vi "Loop_SM.vi"() -> ()   [LabVIEW 2017, in "Overlords.lvlib"]
uses:
  Overlords.lvlib
  ENUM _Overloard Shooter States.ctl
  VisionSystem/Enum_ Field Targets.ctl
  VisionSystem/VisionSystem.lvlib
  MechamumDrive/Enum_SM Cmd Select.ctl
  MechamumDrive/MechamunDrive.lvlib
  MechamumDrive/Cluster_CMD to SM Data.ctl
  MechamumDrive/Global_CMD to SM Data.vi
  MechamumDrive/Global_SM Out Data.vi
  Globals/Global_Hopper Statis.vi
  Hopper/Hopper System.lvlib
  ENUM_Overloard State.ctl
  ENUM_Overloard Gear States.ctl
  Sonar/Global_HW_Data Out.vi
  Sonar/Sonar.lvlib
  MechamumDrive/Global_HW_Status Out.vi
  Gear/Global_HW_Data Out.vi
  Gear/Gear.lvlib
  ENUM_Overloard Climb States.ctl
  Climber/Global_SM_Data Out.vi
  Climber/Climber.lvlib
  Climber/ENUM_SM Cmd Select.ctl
  Climber/Global_CMD to SM Data.vi
  VisionSystem/Global_CMD Data.vi
  VisionSystem/Cluster_CMD to Vision.ctl
  VisionSystem/Global_Vision Status.vi
  Shooter/Global_CMD to SM Data.vi
  Shooter/Shooter.lvlib
  Shooter/ENUM_CMD Select.ctl
  Shooter/Cluster_CMD to SM Data.ctl
  Globals/Global_CMD to SM Data.vi
  Hopper/ENUM_Firing_State.ctl
  Hopper/Cluster_CMD to SM Data.ctl
  Global_CMD Data.vi
  Global_SM_Data Out.vi
panel:
  in  "stop":bool
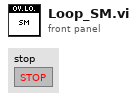
[diagram p1: front panel]
types:
  T1 = typedef "Hopper System.lvlib/ENUM_Firing_State.ctl" = enum16{"No Fireing", "Rapid Fire", "Shotgun Fireing"}
  T2 = typedef "Hopper System.lvlib/Cluster_CMD to SM Data.ctl" = cluster{"Enable Loading":bool, "Disable Loading":bool, "Fireing State":T1, "Time Limit Loading":dbl, "Time Limit Rapid":dbl, "Rapid Fire Shot Limit":i32, "Shotgun Fire Shot Limit":i32}
  T3 = typedef "Shooter.lvlib/ENUM_CMD Select.ctl" = enum16{"Stop", "Manual VBus", "Encoder Hood Only", "Encoder Wheel Only", "Encoder Both"}
  T4 = typedef "Shooter.lvlib/Cluster_CMD to SM Data.ctl" = cluster{"Select":T3, "Wheel VBus":dbl, "Wheel RPM":dbl, "Hood VBus":dbl, "Hood Position":dbl}
  T5 = typedef "MechamunDrive.lvlib/Enum_SM Cmd Select.ctl" = enum16{"No Command", "Halt", "Manual Keep Rotation", "Manual", "Track Front", "Track Rotation", "Track Lateral", "Track Vision Lat", "Track Vision Rot", "Strafe Right", "Strafe Left"}
  T6 = typedef "MechamunDrive.lvlib/Cluster_CMD to SM Data.ctl" = cluster{"CMDMODE":T5, "X":dbl, "Y":dbl, "Rotation":dbl, "Auto Angle":dbl, "Speed Divider":dbl, "Use Gyro":bool, "Target Distance":dbl}
  T7 = typedef "Climber.lvlib/ENUM_SM Cmd Select.ctl" = enum16{"Stop", "Auto Climb", "Manual", "No Command"}
  T8 = typedef "Overlords.lvlib/ENUM_Overloard State.ctl" = enum16{"Idle", "High Shot", "Low Shot", "Place Gear", "Climb"}
  T9 = typedef "Overlords.lvlib/ENUM _Overloard Shooter States.ctl" = enum16{"Startup", "Idle", "Locate Target", "Wait To Be in Position", "Shooting", "Complete"}
  T10 = typedef "VisionSystem.lvlib/Cluster_CMD to Vision.ctl" = cluster{"CMD_Target":T11}
  T11 = typedef "VisionSystem.lvlib/Enum_ Field Targets.ctl" = enum16{"Boiler (USB 0)", "Rope (USB 1)"}
  T12 = typedef "Overlords.lvlib/ENUM_Overloard Gear States.ctl" = enum16{"Startup", "Idle", "Detect Target", "Verticle Track (Sonar)", "Encoder Setup", "Verticle Track (Encoder)", "Gear Present", "Gear Present Counter", "Verticle Backword Track", "Complete"}
  T13 = typedef "Overlords.lvlib/ENUM_Overloard Climb States.ctl" = enum16{"Startup", "Idle", "Check Time", "Check Statis", "Complete"}
  T14 = typedef "Overlords.lvlib/Cluster_CMD to SM Data.ctl" = cluster{"Overloard State":T8, "Match Info":T15, "Firing State":T1, "Gear wait till pullback (seconds)":dbl}
  T15 = typedef "WPI_DriverStationMatch Info.ctl" = cluster{"Autonomous Elapsed Seconds":dbl, "TeleOp Elapsed Seconds":dbl, "Disabled Elapsed Seconds":dbl, "Visited Autonomous":bool, "Visited TeleOp":bool, "Visited Disabled":bool, "Autonomous Settings":cluster{"Autonomous Style":enum16{"Iterative", "Independent"}, "VI Refnum":refnum<vi>}}
  T16 = typedef "Overlords.lvlib/Cluster_SM Status.ctl" = cluster{"Task Complete":bool, "Current Overlord State":T8, "Wanted State":T8, "Overloard Shooter States":T9, "Overlord Gear State":T12, "Overlord Climber State":T13}
  T17 = typedef "Climber.lvlib/Cluster_Cmd to SM Data.ctl" = cluster{"Climber Command Mode":T7}
  T18 = typedef "VisionSystem.lvlib/Cluster_Vision Status.ctl" = cluster{"Target Found":bool, "Target":T11, "Pixels to Center":dbl, "Vision Distance Center (in)":dbl, "Angle Distance Center (in)":dbl}
  T19 = typedef "MechamunDrive.lvlib/Cluster_SM Status.ctl" = cluster{"Drive Cmd":T5, "Complete":bool}
  T20 = typedef "MechamunDrive.lvlib/Cluster_HW Status.ctl" = cluster{"BL":T21, "BR":T21, "FL":T21, "FR":T21}
  T21 = typedef "Cluster_SRX Status With Encoder.ctl" = cluster{"VBus ":dbl, "Module Enabled":bool, "Closed Loop Error":dbl, "Sensor Pos":dbl, "Sensor Vel":dbl, "Current":dbl, "Brake is Enabled":bool, "Encoder Pos":dbl, "Encoder Vel":dbl, " APin":bool, "B Pin":bool, "Bat Voltage":dbl, "Profile Slot":dbl}
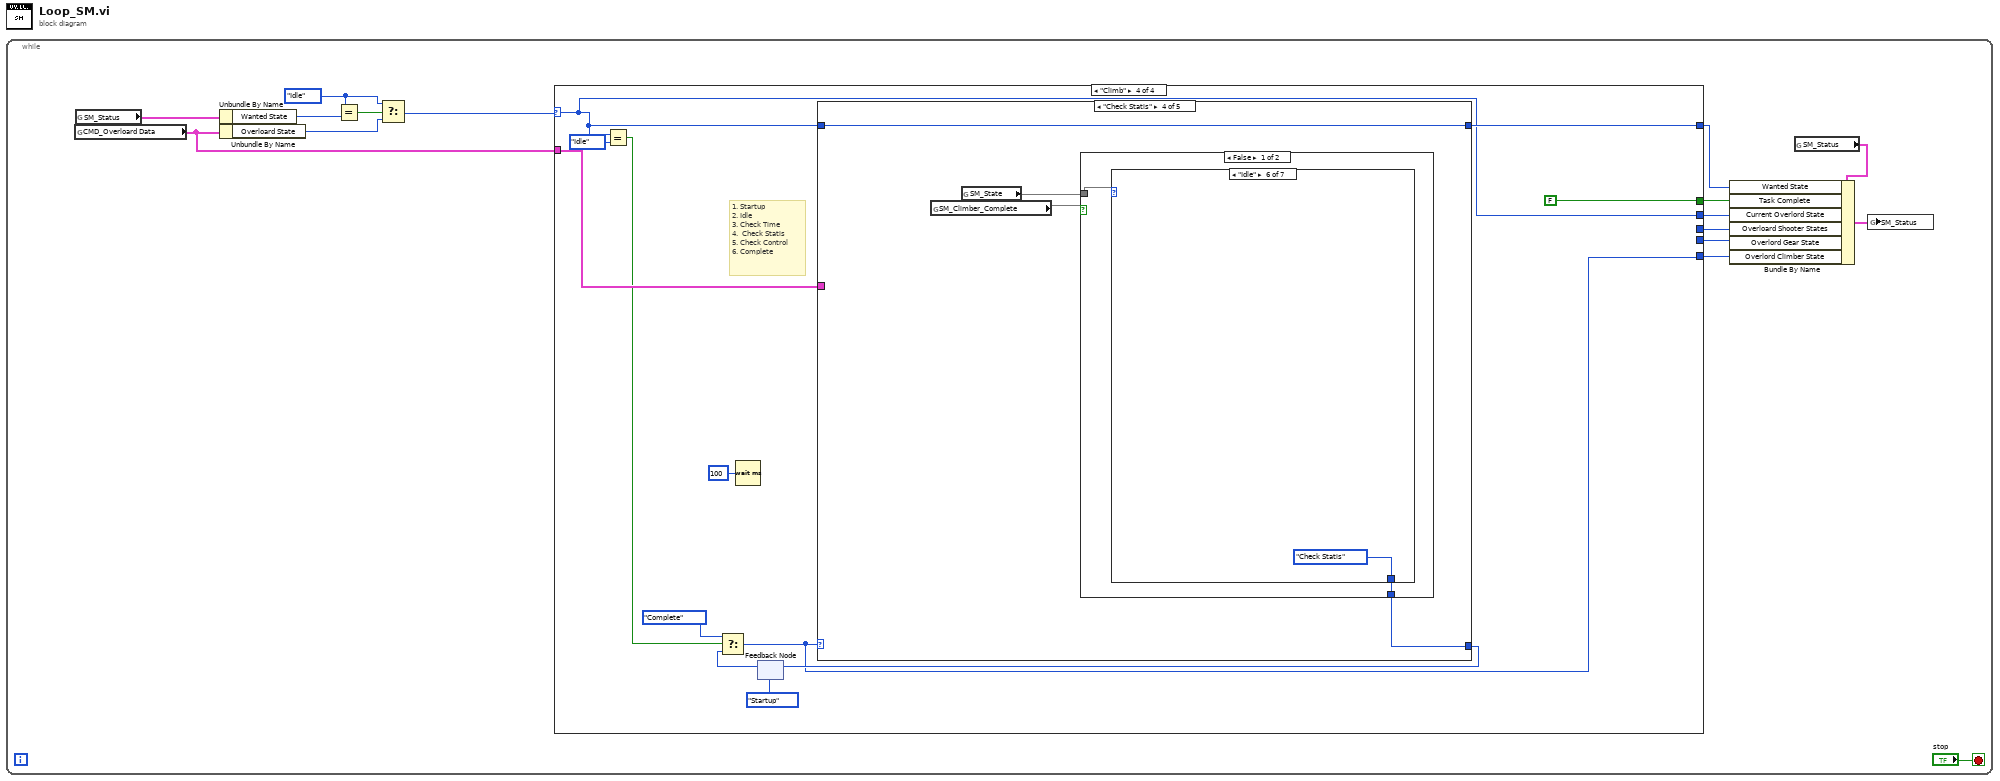
[diagram p0: block diagram]
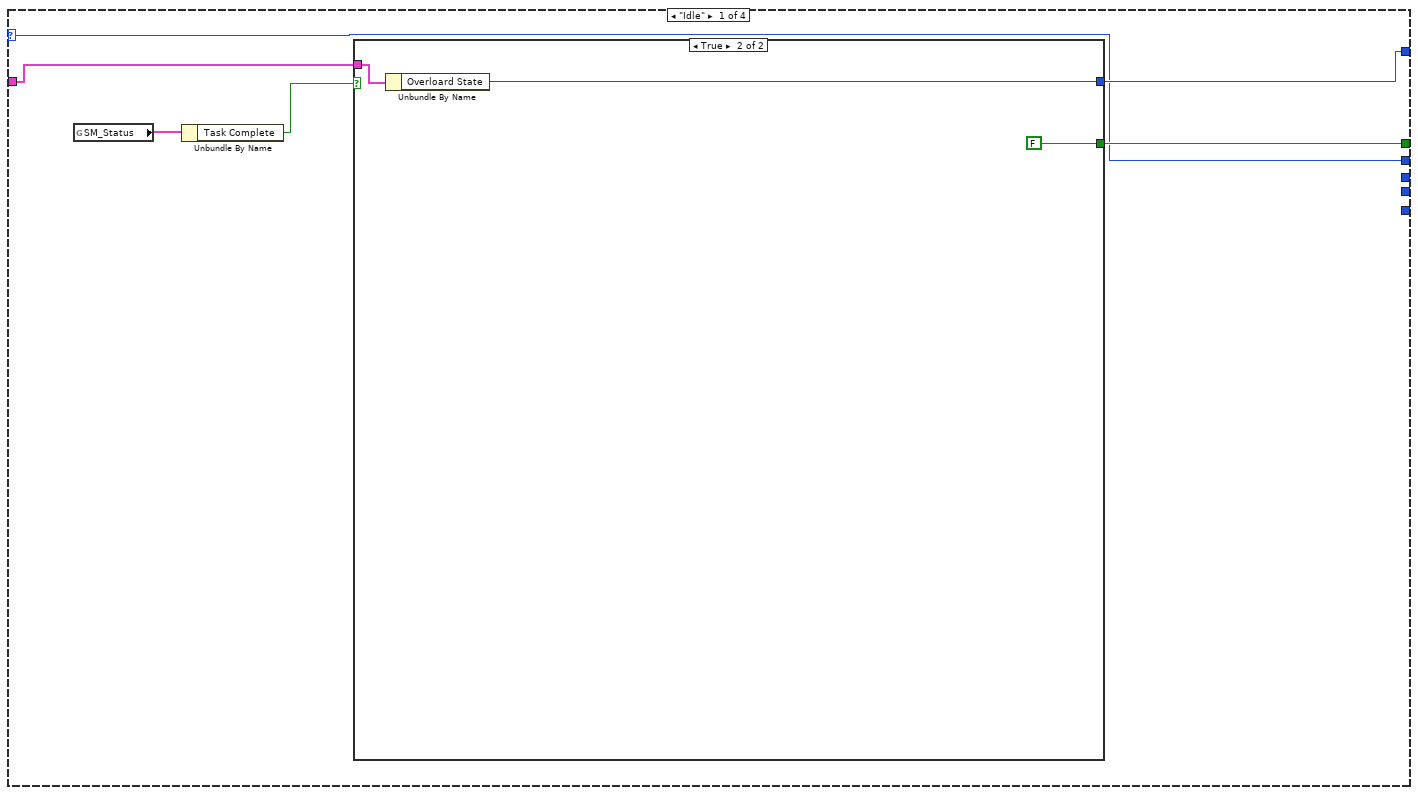
[diagram p2: hidden frame]
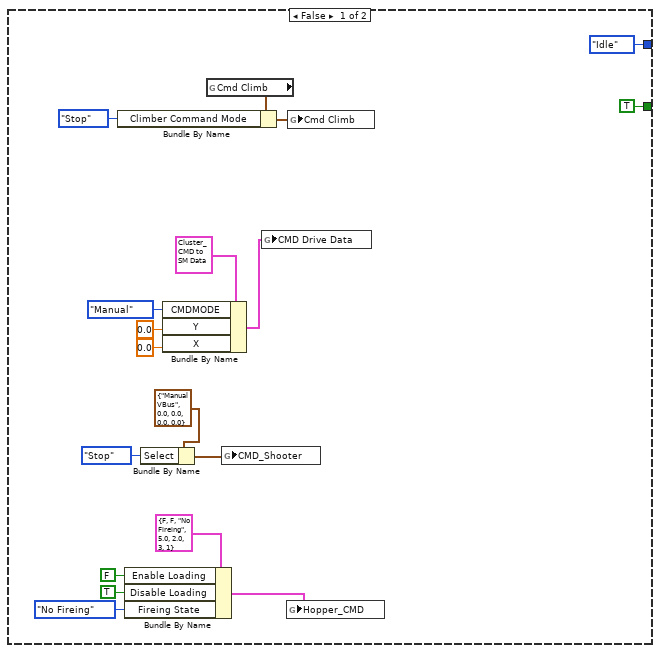
[diagram p3: hidden frame]
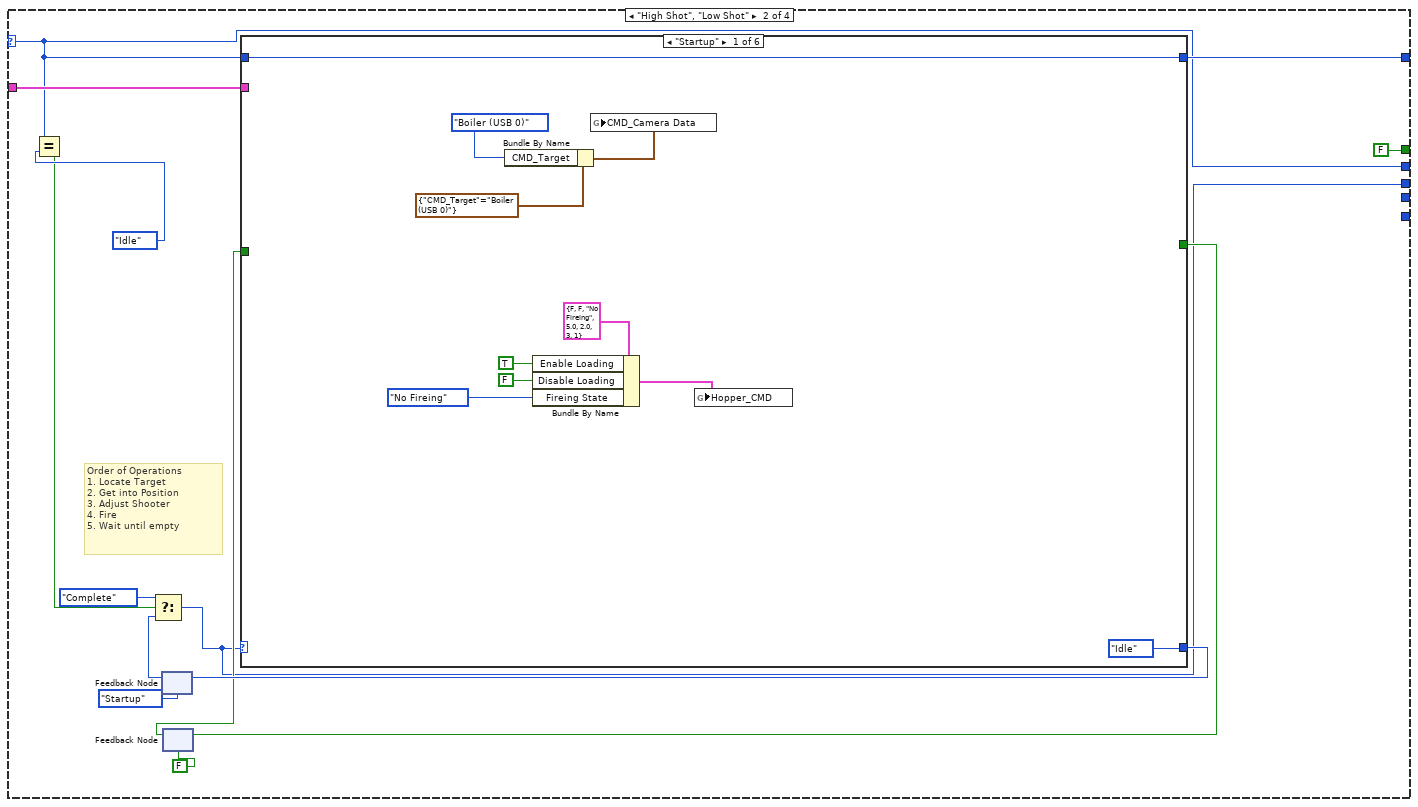
[diagram p4: hidden frame]
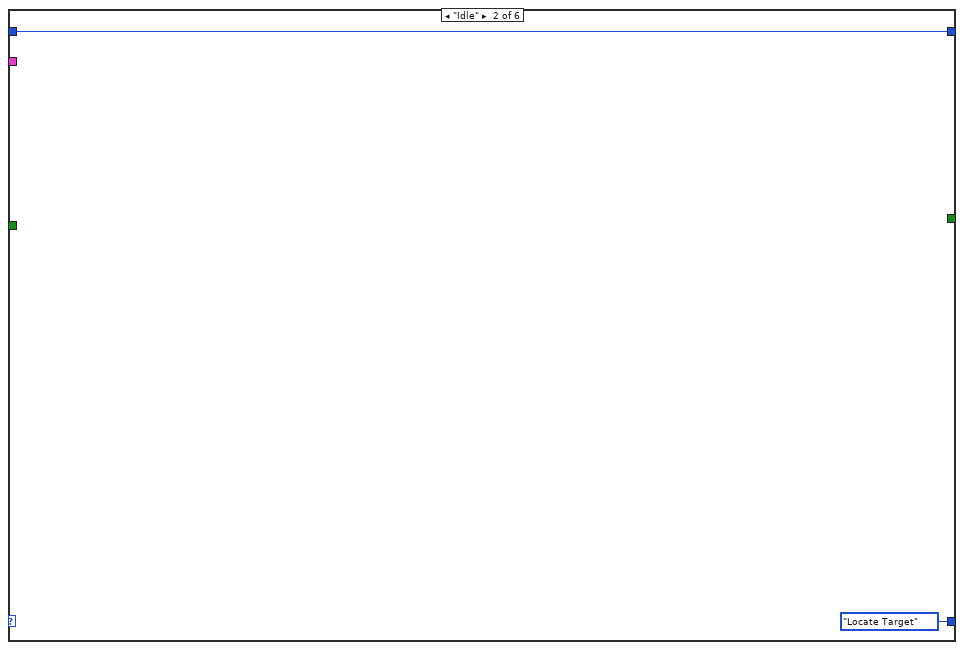
[diagram p5: hidden frame]
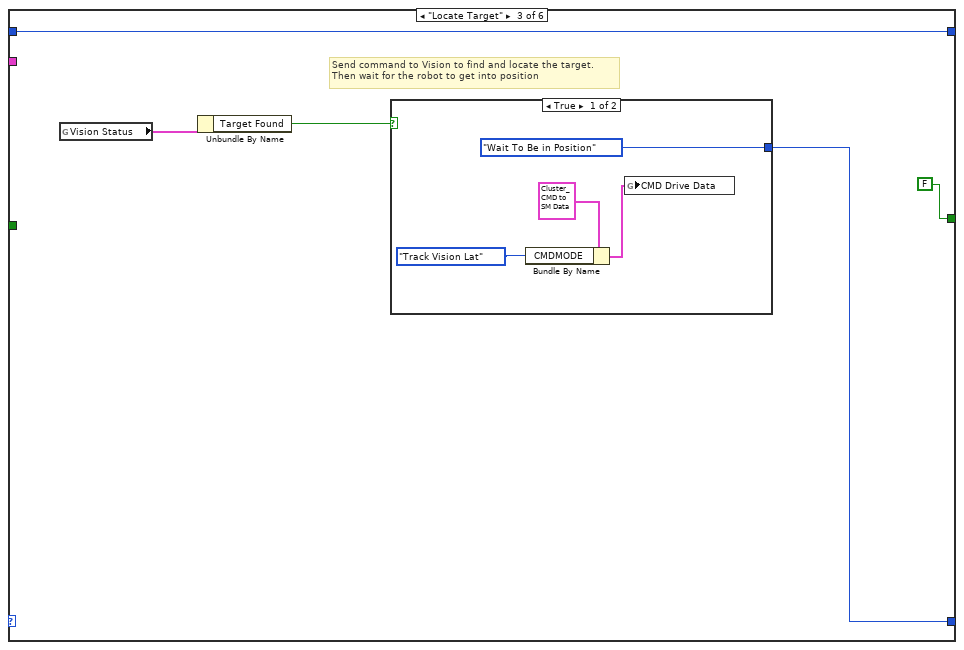
[diagram p6: hidden frame]
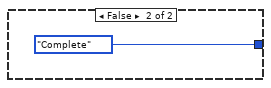
[diagram p7: hidden frame]
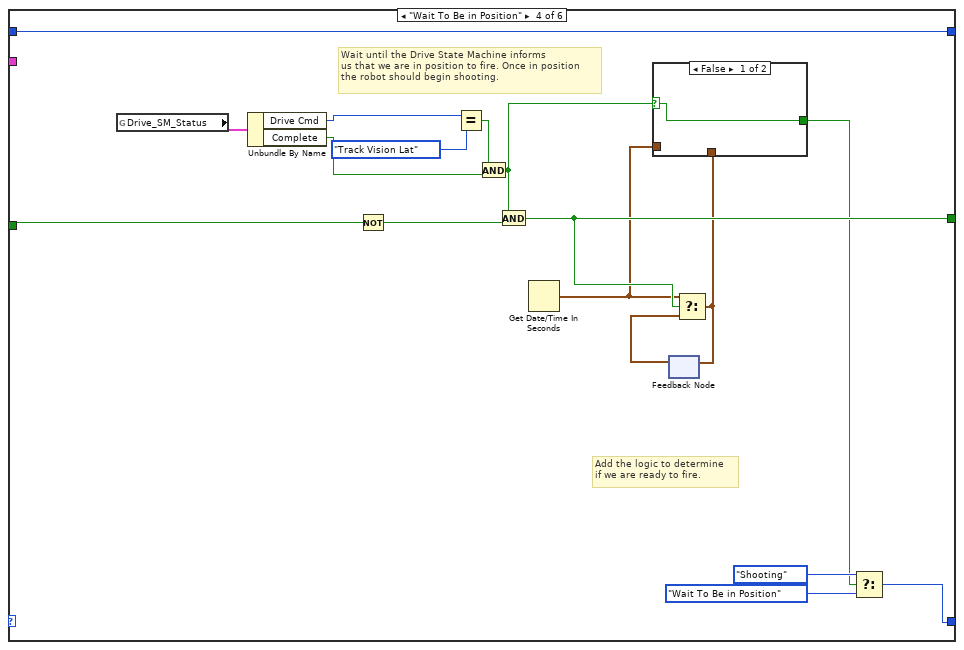
[diagram p8: hidden frame]
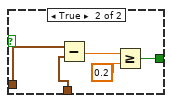
[diagram p9: hidden frame]
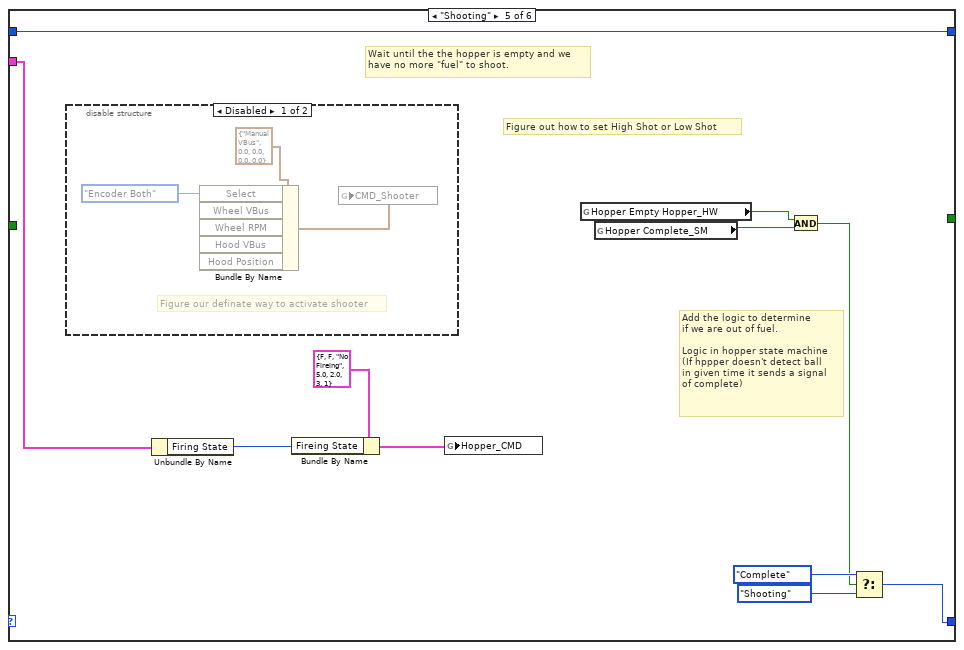
[diagram p10: hidden frame]
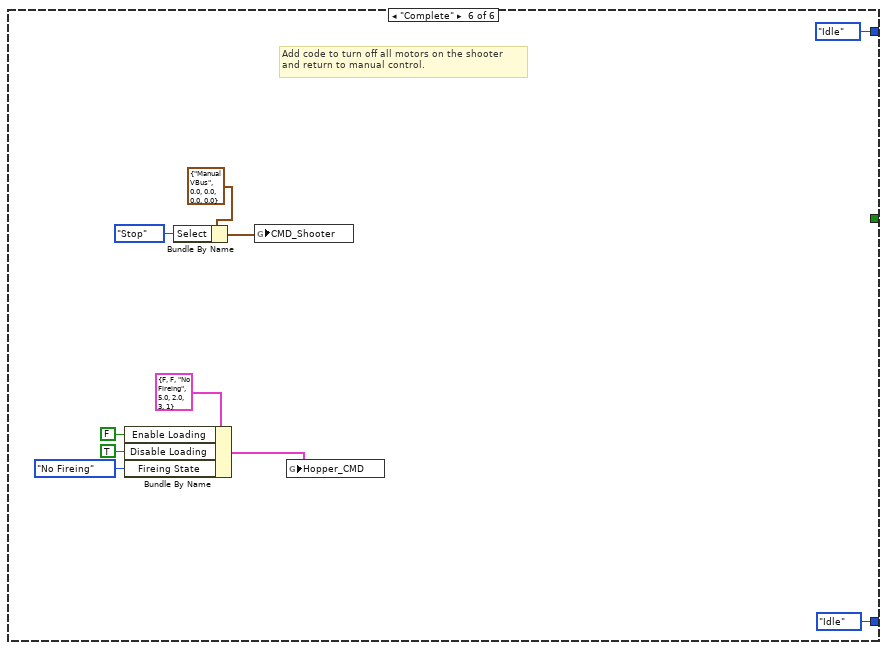
[diagram p12: hidden frame]
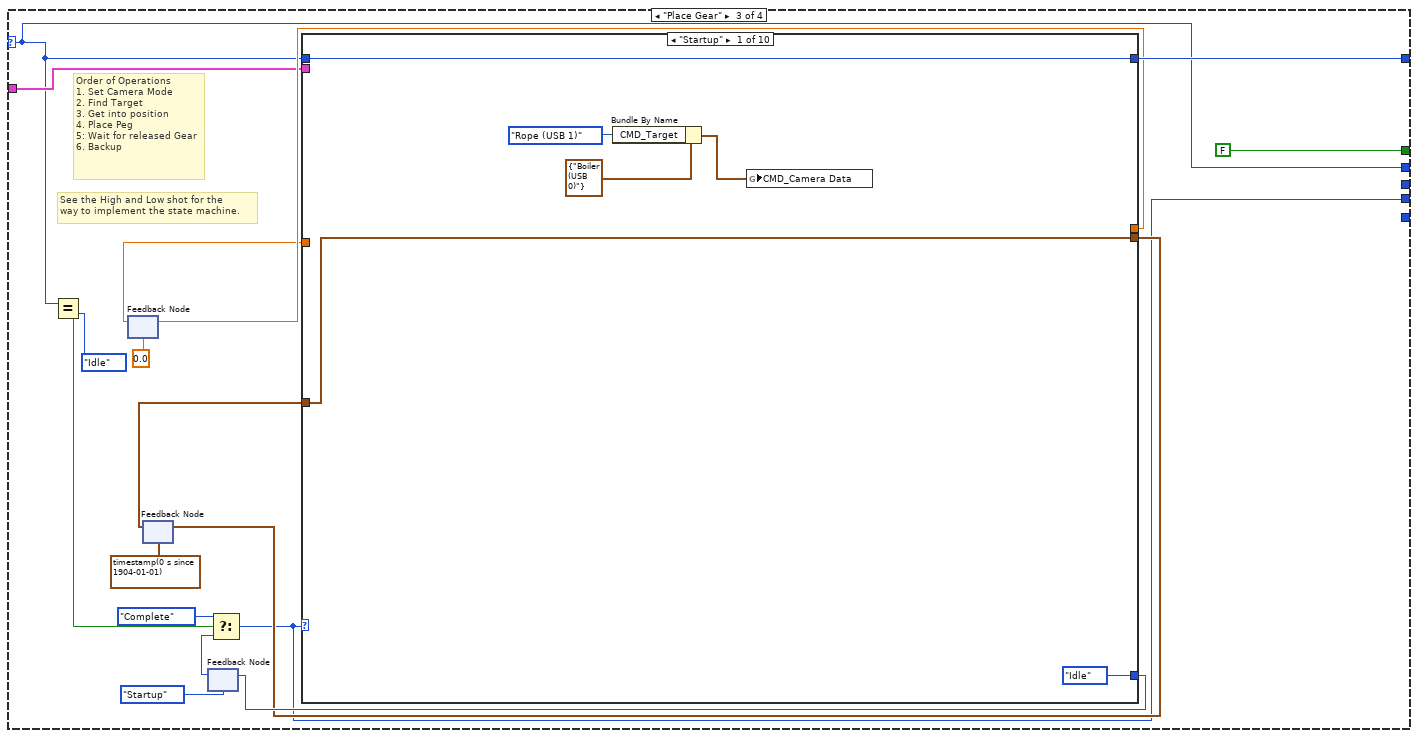
[diagram p13: hidden frame]
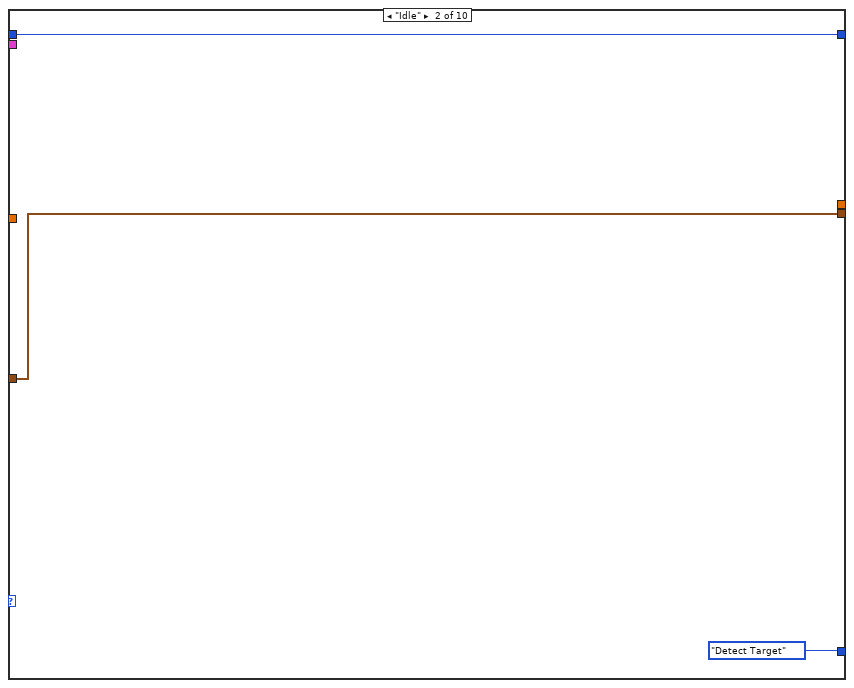
[diagram p14: hidden frame]
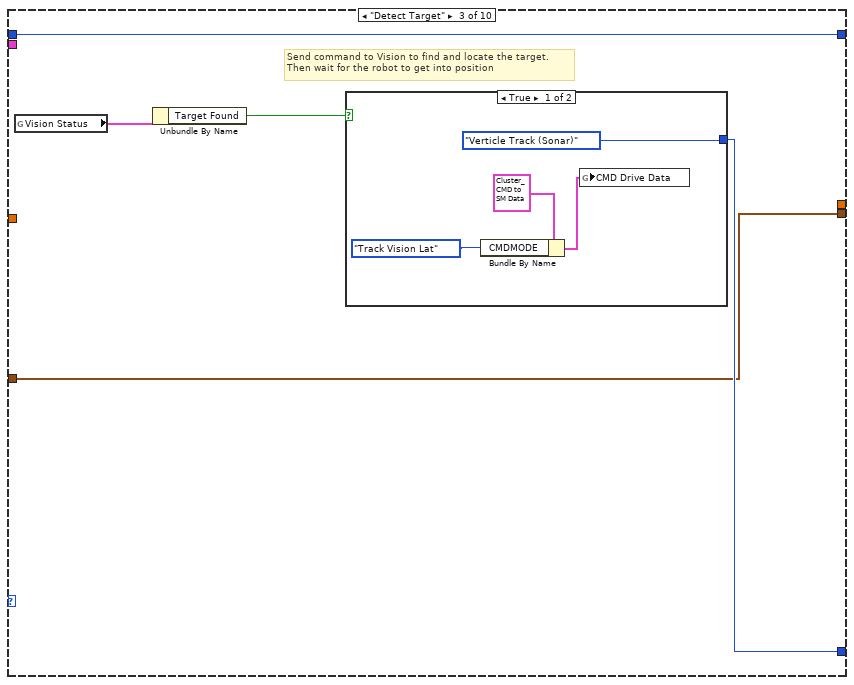
[diagram p15: hidden frame]
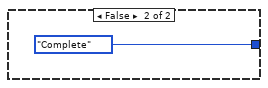
[diagram p16: hidden frame]
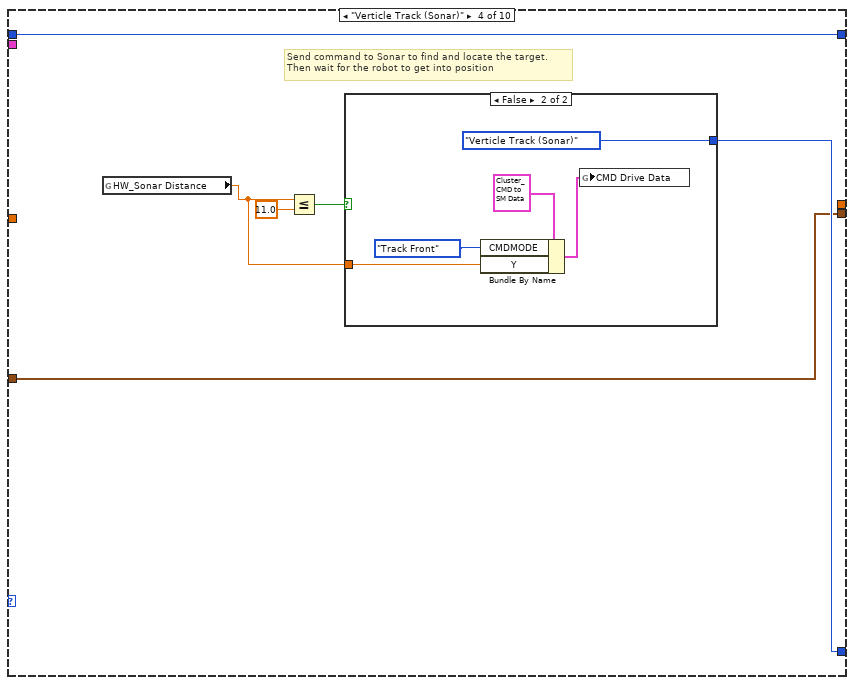
[diagram p17: hidden frame]
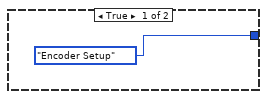
[diagram p18: hidden frame]
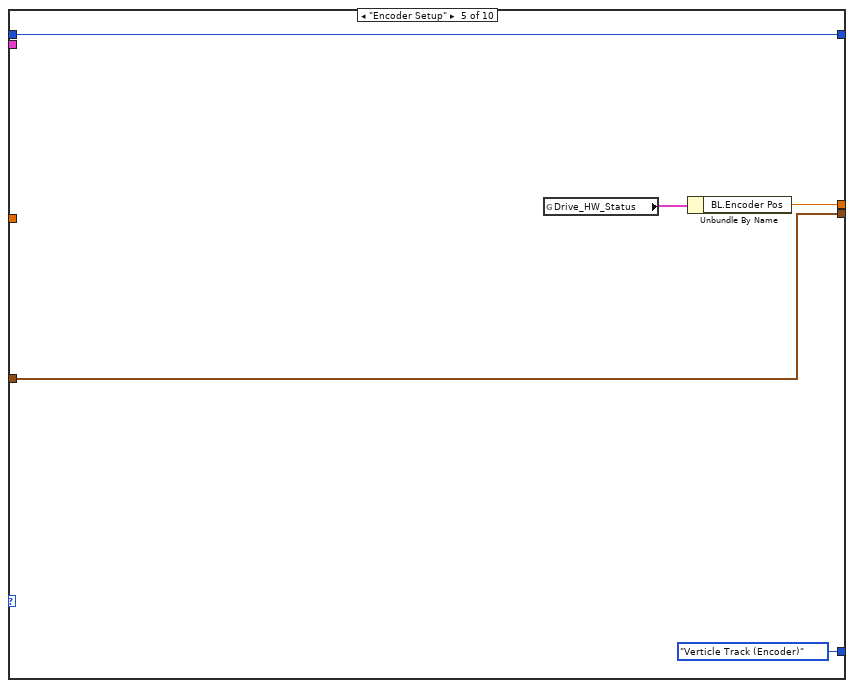
[diagram p19: hidden frame]
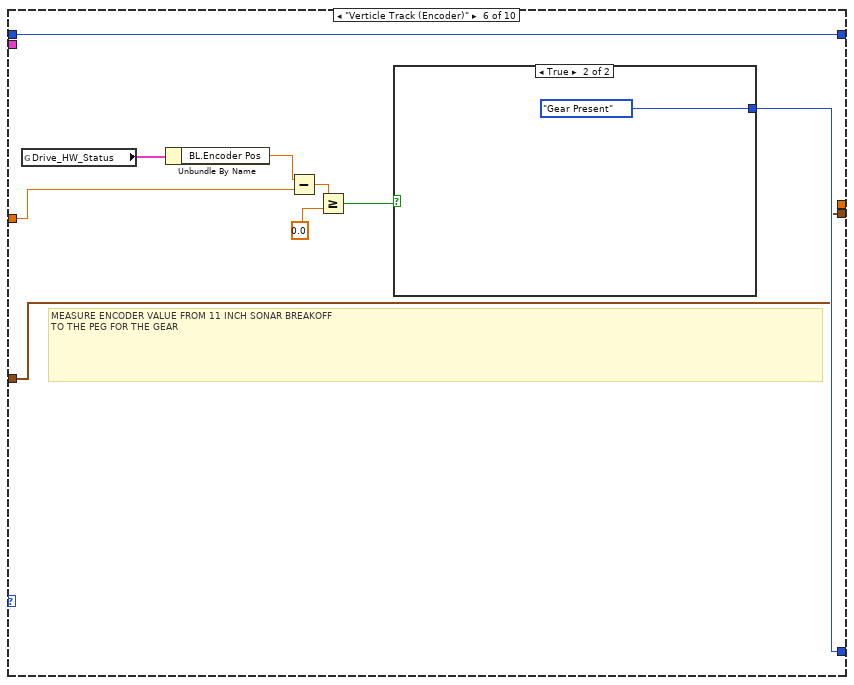
[diagram p20: hidden frame]
diagram:
  n1 = while {
    stop <- "stop" stop-if-true
    w10 = ENUM_Overloard_State."Idle" ("x")
    n2 = global read "Global_CMD Data.vi" "CMD_Overloard Data"() -> (w16:T14)
    n3 = global read "Global_SM_Data Out.vi" "SM_Status"() -> (w13:T16)
    n4 = Unbundle By Name(w13) -> ("Wanted State"=w12:T8)
    n5 = Unbundle By Name(w16) -> ("Overloard State"=w9:T8)
    n6 = Equal?(x=w10, y=w12) -> (x = y?=w11:bool)
    n7 = Select(t=w10, s=w11, f=w9) -> (s? t:f=w8:T8)
    n8 = case shown="\"Climb\"" w8 {
      selector: w8 -> [w17 w45 w128 w227]
      tunnel: [w18 w55 w140 w234] -> w14
      tunnel: w16 -> [w19 w49 w132 w231]
      tunnel: [w22 FALSE FALSE FALSE] -> w15
      tunnel: [w17 w45 w128 w227] -> w7
      tunnel: [_ w44 _ _] -> w6
      tunnel: [_ _ w127 _] -> w5
      tunnel: [_ _ _ w226] -> w4
      frame "Idle" {
        n9 = global read "Global_SM_Data Out.vi" "SM_Status"() -> (w21:T16)
        n10 = Unbundle By Name(w21) -> ("Task Complete"=w20:bool)
        n11 = case shown="True" w20 {
          tunnel: [TRUE FALSE] -> w22
          tunnel: w19 -> [_ w42]
          tunnel: [ENUM_Overloard_State."Idle" ("Overloard State") w41] -> w18
          frame False {
            n12 = Bundle By Name(cluster=T2 {"Enable Loading"=FALSE, "Disable Loading"=FALSE, "Fireing State"=enum."No Fireing", "Time Limit Loading"=5.0, "Time Limit Rapid"=2.0, "Rapid Fire Shot Limit"=3, "Shotgun Fire Shot Limit"=1} ("Hopper_CMD"), "Enable Loading"=FALSE, "Disable Loading"=TRUE, "Fireing State"=ENUM_Firing_State."No Fireing") -> (w27:T2)
            n13 = Bundle By Name(cluster=T4 {"Select"=enum."Manual VBus", "Wheel VBus"=0.0, "Wheel RPM"=0.0, "Hood VBus"=0.0, "Hood Position"=0.0} ("CMD_Shooter"), "Select"=ENUM_CMD_Select."Stop") -> (w29:T4)
            n14 = Bundle By Name(cluster=T6 {"CMDMODE"=enum."No Command", "X"=0.0, "Y"=0.0, "Rotation"=0.0, "Auto Angle"=0.0, "Speed Divider"=0.0, "Use Gyro"=FALSE, "Target Distance"=0.0} ("Drive Data"), "CMDMODE"=Enum_SM_Cmd_Select."Manual", "Y"=0.0, "X"=0.0) -> (w34:T6)
            n15 = global read "Global_CMD to SM Data.vi" "Cmd Climb"() -> (w37:T17)
            n16 = Bundle By Name(cluster=w37, "Climber Command Mode"=ENUM_SM_Cmd_Select."Stop") -> (w38:T17)
            n17 = global write "Global_CMD to SM Data.vi" "CMD_Shooter"(w29) -> ()
            n18 = global write "Global_CMD to SM Data.vi" "CMD Drive Data"(w34) -> ()
            n19 = global write "Global_CMD to SM Data.vi" "Hopper_CMD"(w27) -> ()
            n20 = global write "Global_CMD to SM Data.vi" "Cmd Climb"(w38) -> ()
          }
          frame True {
            n21 = Unbundle By Name(w42) -> ("Overloard State"=w41:T8)
          }
        }
      }
      frame "High Shot", "Low Shot" {
        # "Order of Operations\n1. Locate Target\n2. Get into Position\n3. Adjust Shooter\n4. Fire\n5. Wait until empty"
        n22 = Equal?(x=w45, y=ENUM_Overloard_State."Idle") -> (x = y?=w47:bool)
        n23 = feedback #1(ENUM__Overloard_Shooter_States."Startup" ("Shooter States")) -> (w54:T9)
        n24 = Select(t=ENUM__Overloard_Shooter_States."Complete" ("Shooter States"), s=w47, f=w54) -> (s? t:f=w44:T9)
        n25 = feedback #2(FALSE) -> (w50:bool)
        n26 = case shown="\"Startup\"" w44 {
          tunnel: [ENUM__Overloard_Shooter_States."Idle" ("Shooter States") ENUM__Overloard_Shooter_States."Locate Target" ("Shooter States") w71 w95 w112 ENUM__Overloard_Shooter_States."Idle" ("Shooter States")] -> w57
          tunnel: w45 -> [w67 w69 w74 w96 w113 _]
          tunnel: [w67 w69 w74 w96 w113 ENUM_Overloard_State."Idle" ("Teleop State")] -> w55
          tunnel: [_ _ FALSE w84 _ _] -> w52
          tunnel: w50 -> [_ _ _ w87 _ _]
          tunnel: w49 -> [_ _ _ _ w103 _]
          frame "Startup" {
            n27 = Bundle By Name(cluster=T10 {"CMD_Target"=enum."Boiler (USB 0)"} ("CMD_Camera Data"), "CMD_Target"=Enum__Field_Targets."Boiler (USB 0)" ("CMD_Vision Target")) -> (w63:T10)
            n28 = Bundle By Name(cluster=T2 {"Enable Loading"=FALSE, "Disable Loading"=FALSE, "Fireing State"=enum."No Fireing", "Time Limit Loading"=5.0, "Time Limit Rapid"=2.0, "Rapid Fire Shot Limit"=3, "Shotgun Fire Shot Limit"=1} ("Hopper_CMD"), "Enable Loading"=TRUE, "Disable Loading"=FALSE ("Enable Loading"), "Fireing State"=ENUM_Firing_State."No Fireing") -> (w62:T2)
            n29 = global write "Global_CMD Data.vi" "CMD_Camera Data"(w63) -> ()
            n30 = global write "Global_CMD to SM Data.vi" "Hopper_CMD"(w62) -> ()
          }
          frame "Idle" {
          }
          frame "Locate Target" {
            # "Send command to Vision to find and locate the target.\nThen wait for the robot to get into position"
            n31 = global read "Global_Vision Status.vi" "Vision Status"() -> (w73:T18)
            n32 = Unbundle By Name(w73) -> ("Target Found"=w72:bool)
            n33 = case shown="True" w72 {
              tunnel: [ENUM__Overloard_Shooter_States."Wait To Be in Position" ("Shooter States") ENUM__Overloard_Shooter_States."Complete" ("Shooter States")] -> w71
              frame True {
                n34 = Bundle By Name(cluster=T6 {"CMDMODE"=enum."No Command", "X"=0.0, "Y"=0.0, "Rotation"=0.0, "Auto Angle"=0.0, "Speed Divider"=0.0, "Use Gyro"=FALSE, "Target Distance"=0.0} ("Drive Data"), "CMDMODE"=Enum_SM_Cmd_Select."Track Vision Lat") -> (w76:T6)
                n35 = global write "Global_CMD to SM Data.vi" "CMD Drive Data"(w76) -> ()
              }
              frame False {
              }
            }
          }
          frame "Wait To Be in Position" {
            # "Add the logic to determine\nif we are ready to fire."
            # "Wait until the Drive State Machine informs\nus that we are in position to fire. Once in position\nthe robot should begin shooting."
            n36 = global read "Global_SM Out Data.vi" "Drive_SM_Status"() -> (w92:T19)
            n37 = Unbundle By Name(w92) -> ("Drive Cmd"=w91:T5, "Complete"=w86:bool)
            n38 = Not(x=w87) -> (.not. x?=w88:bool)
            n39 = Equal?(x=w91, y=Enum_SM_Cmd_Select."Track Vision Lat") -> (x = y?=w89:bool)
            n40 = And(x=w89, y=w86) -> (x .and. y?=w83:bool)
            n41 = And(x=w83, y=w88) -> (x .and. y?=w84:bool)
            n42 = Get Date/Time In Seconds() -> (seconds since 1Jan1904=w81:timestamp)
            n43 = feedback #3() -> (w85:timestamp)  [unwired: 1 in]
            n44 = Select(t=w81, s=w84, f=w85) -> (s? t:f=w82:timestamp)
            n45 = case shown="False" w83 {
              selector: w83 -> [w97 _]
              tunnel: w82 -> [_ w101]
              tunnel: w81 -> [_ w102]
              tunnel: [w97 w98] -> w80
              frame False {
              }
              frame True {
                n46 = Subtract(x=w102, y=w101) -> (x-y=w100:dbl)
                n47 = Greater Or Equal?(x=w100, y=0.2) -> (x >= y?=w98:bool)
              }
            }
            n48 = feedback-in #3(w82) -> ()
            n49 = Select(t=ENUM__Overloard_Shooter_States."Shooting" ("Shooter States"), s=w80, f=ENUM__Overloard_Shooter_States."Wait To Be in Position" ("Shooter States")) -> (s? t:f=w95:T9)
          }
          frame "Shooting" {
            # "Figure out how to set High Shot or Low Shot"
            # "Add the logic to determine\nif we are out of fuel.\n\nLogic in hopper state machine\n(If hppper doesn't detect ball\nin given time it sends a signal\nof complete)"
            # "Wait until the the hopper is empty and we\nhave no more \"fuel\" to shoot."
            n50 = disable-structure shown="Disabled" {
              frame Disabled {
                # "Figure our definate way to activate shooter"
                n51 = Bundle By Name(cluster=T4 {"Select"=enum."Manual VBus", "Wheel VBus"=0.0, "Wheel RPM"=0.0, "Hood VBus"=0.0, "Hood Position"=0.0} ("CMD_Shooter"), "Select"=ENUM_CMD_Select."Encoder Both") -> (w115:T4)  [unwired: 4 in]
                n52 = global write "Global_CMD to SM Data.vi" "CMD_Shooter"(w115) -> ()
              }
              frame Enabled {
              }
            }
            n53 = Unbundle By Name(w103) -> ("Firing State"=w104:T1)
            n54 = Bundle By Name(cluster=T2 {"Enable Loading"=FALSE, "Disable Loading"=FALSE, "Fireing State"=enum."No Fireing", "Time Limit Loading"=5.0, "Time Limit Rapid"=2.0, "Rapid Fire Shot Limit"=3, "Shotgun Fire Shot Limit"=1} ("Hopper_CMD"), "Fireing State"=w104) -> (w106:T2)
            n55 = global write "Global_CMD to SM Data.vi" "Hopper_CMD"(w106) -> ()
            n56 = global read "Global_Hopper Statis.vi" "Hopper Empty Hopper_HW"() -> (w109:bool)
            n57 = global read "Global_Hopper Statis.vi" "Hopper Complete_SM"() -> (w108:bool)
            n58 = And(x=w109, y=w108) -> (x .and. y?=w107:bool)
            n59 = Select(t=ENUM__Overloard_Shooter_States."Complete" ("Shooter States"), s=w107, f=ENUM__Overloard_Shooter_States."Shooting" ("Shooter States")) -> (s? t:f=w112:T9)
          }
          frame "Complete" {
            # "Add code to turn off all motors on the shooter\nand return to manual control."
            n60 = Bundle By Name(cluster=T2 {"Enable Loading"=FALSE, "Disable Loading"=FALSE, "Fireing State"=enum."No Fireing", "Time Limit Loading"=5.0, "Time Limit Rapid"=2.0, "Rapid Fire Shot Limit"=3, "Shotgun Fire Shot Limit"=1} ("Hopper_CMD"), "Enable Loading"=FALSE, "Disable Loading"=TRUE, "Fireing State"=ENUM_Firing_State."No Fireing") -> (w121:T2)
            n61 = Bundle By Name(cluster=T4 {"Select"=enum."Manual VBus", "Wheel VBus"=0.0, "Wheel RPM"=0.0, "Hood VBus"=0.0, "Hood Position"=0.0} ("CMD_Shooter"), "Select"=ENUM_CMD_Select."Stop") -> (w123:T4)
            n62 = global write "Global_CMD to SM Data.vi" "CMD_Shooter"(w123) -> ()
            n63 = global write "Global_CMD to SM Data.vi" "Hopper_CMD"(w121) -> ()
          }
        }
        n64 = feedback-in #1(w57) -> ()
        n65 = feedback-in #2(w52) -> ()
      }
      frame "Place Gear" {
        # "See the High and Low shot for the\nway to implement the state machine."
        # "Order of Operations\n1. Set Camera Mode\n2. Find Target\n3. Get into position \n4. Place Peg\n5: Wait for released Gear\n6. Backup"
        n66 = Equal?(x=w128, y=ENUM_Overloard_State."Idle") -> (x = y?=w130:bool)
        n67 = feedback #4(0.0 ("Encoder Pos")) -> (w136:dbl)
        n68 = feedback #5(timestamp(0 s since 1904-01-01) ("seconds since 1Jan1904")) -> (w133:timestamp)
        n69 = feedback #6(ENUM_Overloard_Gear_States."Startup") -> (w142:T12)
        n70 = Select(t=ENUM_Overloard_Gear_States."Complete", s=w130, f=w142) -> (s? t:f=w127:T12)
        n71 = case shown="\"Startup\"" w127 {
          tunnel: [w149 w152 w157 w168 w179 w188 w199 w208 w221 ENUM_Overloard_State."Idle" ("Teleop State")] -> w140
          tunnel: w128 -> [w149 w152 w157 w168 w179 w188 w199 w208 w221 _]
          tunnel: [ENUM_Overloard_Gear_States."Idle" ENUM_Overloard_Gear_States."Detect Target" w154 w167 ENUM_Overloard_Gear_States."Verticle Track (Encoder)" ("t") w181 w197 w206 ENUM_Overloard_Gear_States."Complete" ("t") ENUM_Overloard_Gear_States."Idle" ("t")] -> w139
          tunnel: [_ _ _ _ w176 _ _ _ _ _] -> w138
          tunnel: w136 -> [_ _ _ _ _ w185 _ _ _ _]
          tunnel: [w147 w150 w153 w163 w175 w180 w196 w205 w219 w223] -> w135
          tunnel: w133 -> [w147 w150 w153 w163 w175 w180 _ w205 w219 w223]
          tunnel: w132 -> [_ _ _ _ _ _ _ w204 _ _]
          frame "Startup" {
            n72 = Bundle By Name(cluster=T10 {"CMD_Target"=enum."Boiler (USB 0)"} ("CMD_Camera Data"), "CMD_Target"=Enum__Field_Targets."Rope (USB 1)" ("CMD_Vision Target")) -> (w144:T10)
            n73 = global write "Global_CMD Data.vi" "CMD_Camera Data"(w144) -> ()
          }
          frame "Idle" {
          }
          frame "Detect Target" {
            # "Send command to Vision to find and locate the target.\nThen wait for the robot to get into position"
            n74 = global read "Global_Vision Status.vi" "Vision Status"() -> (w156:T18)
            n75 = Unbundle By Name(w156) -> ("Target Found"=w155:bool)
            n76 = case shown="True" w155 {
              tunnel: [ENUM_Overloard_Gear_States."Verticle Track (Sonar)" ("t") ENUM_Overloard_Gear_States."Complete" ("t")] -> w154
              frame True {
                n77 = Bundle By Name(cluster=T6 {"CMDMODE"=enum."No Command", "X"=0.0, "Y"=0.0, "Rotation"=0.0, "Auto Angle"=0.0, "Speed Divider"=0.0, "Use Gyro"=FALSE, "Target Distance"=0.0} ("Drive Data"), "CMDMODE"=Enum_SM_Cmd_Select."Track Vision Lat") -> (w160:T6)
                n78 = global write "Global_CMD to SM Data.vi" "CMD Drive Data"(w160) -> ()
              }
              frame False {
              }
            }
          }
          frame "Verticle Track (Sonar)" {
            # "Send command to Sonar to find and locate the target.\nThen wait for the robot to get into position"
            n79 = global read "Global_HW_Data Out.vi" "HW_Sonar Distance"() -> (w164:dbl)
            n80 = Less Or Equal?(x=w164, y=11.0) -> (x <= y?=w166:bool)
            n81 = case shown="False" w166 {
              tunnel: [ENUM_Overloard_Gear_States."Encoder Setup" ("t") ENUM_Overloard_Gear_States."Verticle Track (Sonar)" ("t")] -> w167
              tunnel: w164 -> [_ w170]
              frame True {
              }
              frame False {
                n82 = Bundle By Name(cluster=T6 {"CMDMODE"=enum."No Command", "X"=0.0, "Y"=0.0, "Rotation"=0.0, "Auto Angle"=0.0, "Speed Divider"=0.0, "Use Gyro"=FALSE, "Target Distance"=0.0} ("Drive Data"), "CMDMODE"=Enum_SM_Cmd_Select."Track Front", "Y"=w170) -> (w172:T6)
                n83 = global write "Global_CMD to SM Data.vi" "CMD Drive Data"(w172) -> ()
              }
            }
          }
          frame "Encoder Setup" {
            n84 = global read "Global_HW_Status Out.vi" "Drive_HW_Status"() -> (w178:T20)
            n85 = Unbundle By Name(w178) -> ("BL.Encoder Pos"=w176:dbl)
          }
          frame "Verticle Track (Encoder)" {
            # "MEASURE ENCODER VALUE FROM 11 INCH SONAR BREAKOFF\nTO THE PEG FOR THE GEAR"
            n86 = global read "Global_HW_Status Out.vi" "Drive_HW_Status"() -> (w187:T20)
            n87 = Unbundle By Name(w187) -> ("BL.Encoder Pos"=w186:dbl)
            n88 = Subtract(x=w186, y=w185) -> (x-y=w184:dbl)
            n89 = Greater Or Equal?(x=w184, y=0.0) -> (x >= y?=w182:bool)
            n90 = case shown="True" w182 {
              tunnel: [ENUM_Overloard_Gear_States."Verticle Track (Encoder)" ("t") ENUM_Overloard_Gear_States."Gear Present" ("t")] -> w181
              frame False {
                n91 = Bundle By Name(cluster=T6 {"CMDMODE"=enum."No Command", "X"=0.0, "Y"=0.0, "Rotation"=0.0, "Auto Angle"=0.0, "Speed Divider"=0.0, "Use Gyro"=FALSE, "Target Distance"=0.0} ("Drive Data"), "CMDMODE"=Enum_SM_Cmd_Select."Track Front", "Target Distance"=1.0, "Speed Divider"=3.0) -> (w193:T6)
                n92 = global write "Global_CMD to SM Data.vi" "CMD Drive Data"(w193) -> ()
              }
              frame True {
              }
            }
          }
          frame "Gear Present" {
            # "Gear Lib removed"
            n93 = global read "Global_HW_Data Out.vi" "HW_Gear Present"() -> (w198:bool)
            n94 = case shown="True" w198 {
              tunnel: [ENUM_Overloard_Gear_States."Gear Present" ("t") ENUM_Overloard_Gear_States."Gear Present Counter" ("t")] -> w197
              tunnel: [timestamp(0 s since 1904-01-01) ("seconds since 1Jan1904") w202] -> w196
              frame True {
              }
              frame False {
                n95 = Get Date/Time In Seconds() -> (seconds since 1Jan1904=w202:timestamp)
              }
            }
          }
          frame "Gear Present Counter" {
            n96 = global read "Global_HW_Data Out.vi" "HW_Gear Present"() -> (w207:bool)
            n97 = case shown="False" w207 {
              tunnel: [w211 ENUM_Overloard_Gear_States."Gear Present" ("t")] -> w206
              tunnel: w205 -> [w214 _]
              tunnel: w204 -> [w210 _]
              frame False {
                n98 = Unbundle By Name(w210) -> ("Gear wait till pullback (seconds)"=w209:dbl)
                n99 = Get Date/Time In Seconds() -> (seconds since 1Jan1904=w215:timestamp)
                n100 = Subtract(x=w215, y=w214) -> (x-y=w213:dbl)
                n101 = Greater Or Equal?(x=w213, y=w209) -> (x >= y?=w212:bool)
                n102 = case shown="True" w212 {
                  tunnel: [ENUM_Overloard_Gear_States."Verticle Backword Track" ("t") ENUM_Overloard_Gear_States."Gear Present Counter" ("t")] -> w211
                  frame True {
                  }
                  frame False {
                  }
                }
              }
              frame True {
              }
            }
          }
          frame "Verticle Backword Track" {
            # "Track Backward removed from drive commands"
          }
          frame "Complete" {
          }
        }
        n103 = feedback-in #4(w138) -> ()
        n104 = feedback-in #5(w135) -> ()
        n105 = feedback-in #6(w139) -> ()
      }
      frame "Climb" {
        # "1. Startup\n2. Idle\n3. Check Time\n4.  Check Statis\n5. Check Control\n6. Complete"
        n106 = Equal?(x=w227, y=ENUM_Overloard_State."Idle") -> (x = y?=w229:bool)
        n107 = Wait (ms)(milliseconds to wait=u32 100) -> ()  [unwired: 1 out]
        n108 = feedback #7(ENUM_Overloard_Climb_States."Startup") -> (w233:T13)
        n109 = Select(t=ENUM_Overloard_Climb_States."Complete", s=w229, f=w233) -> (s? t:f=w226:T13)
        n110 = case shown="\"Check Statis\"" w226 {
          tunnel: [ENUM_Overloard_Climb_States."Startup" ENUM_Overloard_Climb_States."Idle" w242 w249 ENUM_Overloard_Climb_States."Idle"] -> w235
          tunnel: w227 -> [w237 w240 w246 w252 _]
          tunnel: [w237 w240 w246 w252 ENUM_Overloard_State."Idle" ("Teleop State")] -> w234
          tunnel: w231 -> [_ _ w241 _ _]
          frame "Startup" {
          }
          frame "Idle" {
          }
          frame "Check Time" {
            w244 = 105.0  # Second Timer for when Rope goes down in Teleop 135 in Teleop, Rope releases in final 30 seconds
            n111 = Unbundle By Name(w241) -> ("Match Info.TeleOp Elapsed Seconds"=w245:dbl)
            n112 = Greater Or Equal?(x=w245, y=w244) -> (x >= y?=w243:bool)
            n113 = case shown="True" w243 {
              tunnel: [ENUM_Overloard_Climb_States."Check Statis" ENUM_Overloard_Climb_States."Complete"] -> w242
              frame True {
              }
              frame False {
              }
            }
          }
          frame "Check Statis" {
            n114 = global read "Global_SM_Data Out.vi" "SM_Climber_Complete"() -> (w251)
            n115 = global read "Global_SM_Data Out.vi" "SM_State"() -> (w250)
            n116 = case shown="False" w251 {
              tunnel: w250 -> [w254 _]
              tunnel: [w253 ENUM_Overloard_Climb_States."Complete"] -> w249
              frame False {
                n117 = case shown="\"Idle\"" w254 {
                  tunnel: [ENUM_Overloard_Climb_States."Check Statis" ENUM_Overloard_Climb_States."Check Statis" ENUM_Overloard_Climb_States."Check Statis" ENUM_Overloard_Climb_States."Check Statis" ENUM_Overloard_Climb_States."Idle" ENUM_Overloard_Climb_States."Check Statis" ENUM_Overloard_Climb_States."Complete"] -> w253
                  frame "Auto Rope Engage" {
                  }
                  frame "Auto Rope Climb" {
                  }
                  frame "Manual Speed Control" {
                  }
                  frame "No command" {
                  }
                  frame "Startup" {
                  }
                  frame "Idle" {
                  }
                  frame "Shutdown" {
                  }
                }
              }
              frame True {
              }
            }
          }
          frame "Complete" {
            n118 = global read "Global_CMD to SM Data.vi" "Cmd Climb"() -> (w266:T17)
            n119 = Bundle By Name(cluster=w266, "Climber Command Mode"=ENUM_SM_Cmd_Select."Stop") -> (w267:T17)
            n120 = global write "Global_CMD to SM Data.vi" "Cmd Climb"(w267) -> ()
          }
        }
        n121 = feedback-in #7(w235) -> ()
      }
    }
    n122 = global read "Global_SM_Data Out.vi" "SM_Status"() -> (w3:T16)
    n123 = Bundle By Name(cluster=w3, "Wanted State"=w14, "Task Complete"=w15, "Current Overlord State"=w7, "Overloard Shooter States"=w6, "Overlord Gear State"=w5, "Overlord Climber State"=w4) -> (w2:T16)
    n124 = global write "Global_SM_Data Out.vi" "SM_Status"(w2) -> ()
  }
